vi "Enc.vi"(0 "FPGA VI Reference In":refnum<k20>, 1 "steering frame in":refnum<class "NI_Robotics_Steering Frame.lvclass">, 3 "error in":errorcluster) -> (7 "FPGA VI Reference Out":refnum<k20>, 8 "steering frame out":refnum<class "NI_Robotics_Steering Frame.lvclass">, 9 "EnVal":dbl[](array[numeric]), 10 "error out":errorcluster)   [LabVIEW 2019]
uses:
  <vilib>/robotics/Steering/Steering Frame/NI_Robotics_Steering Frame.lvclass
  <vilib>/Utility/error.llb/Error Cluster From Error Code.vi
  <vilib>/rvi/errors/niLvFpgaAdjustHostInterfaceError.vi
  <vilib>/robotics/Steering/Steering Frame/Get Steering Frame Velocity from Motors.vi
  <vilib>/rvi/interface/nirviReadWriteControl/nirviReadWriteControl.xnode
  NiFpgaLv.dll
  <vilib>/rvi/interface/Simulation/niFpgaSimulationCallBeginRW.vi
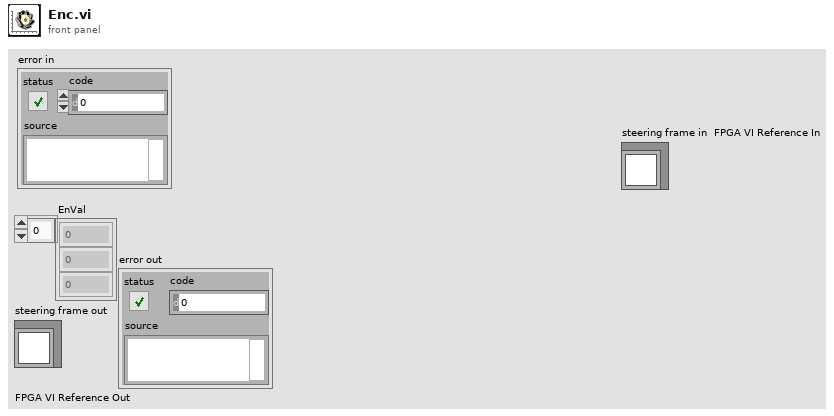
[diagram p1: front panel]
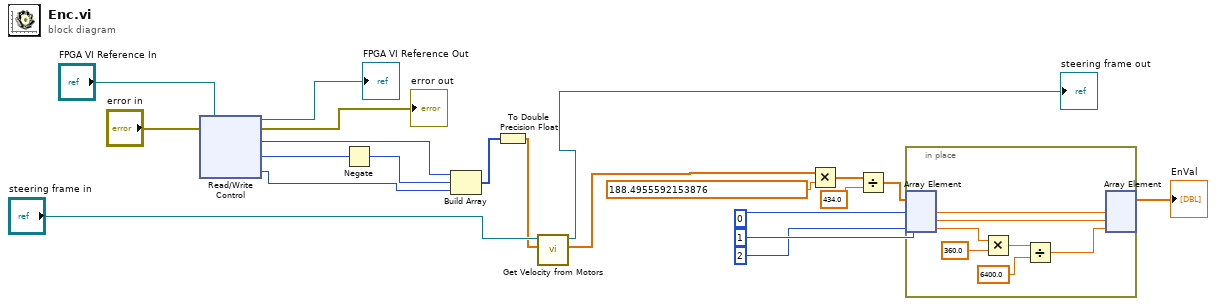
[diagram p0: block diagram]
diagram:
  n1 = xnode "Read/Write Control"("FPGA VI Reference In"="FPGA VI Reference In", "error in"="error in") -> ("FPGA VI Reference Out"=→"FPGA VI Reference Out":refnum<k20>, "error out"=→"error out":errorcluster, "ENC M1"=w4:i32, "ENC M2"=w3:i32, "ENC M3"=w1:i32)
  n2 = Negate(x=w3) -> (-x=w2:i32)
  n3 = Build Array(w4, w2, w1) -> (w21:i32[])
  n4 = To Double Precision Float(number=w21) -> (double precision float=w7:dbl[])
  n5 = call-poly <vilib>:"Get Velocity from Motors.vi"("ccw motor velocity states"=w7, "steering frame in"="steering frame in") -> ("estimated steering frame velocity"=w5:dbl[], "steering frame out"=→"steering frame out":refnum<class "NI_Robotics_Steering Frame.lvclass">)  [unwired: 7 in, 1 out]
  n6 = Multiply(x=w5, y=188.4955592153876) -> (x*y=w17:dbl[])
  n7 = Divide(x=w17, y=434.0 ("x")) -> (x/y=w15:dbl[])
  n8 = in-place {
    n9 = in-place-array #1(w15, 0, 1, 2) -> (w24:dbl, w23:dbl, w22:dbl)
    n10 = Multiply(x=w22, y=360.0) -> (x*y=w27:dbl)
    n11 = Divide(x=w27, y=6400.0) -> (x/y=w25:dbl)
    n12 = in-place-array #1(w24, w23, w25) -> (→"EnVal":dbl[])  [unwired: 3 out]
  }
